vi "DOE Add TC Calibration.vi"(7 "Enum":T1, 10 "TC Coefficients":T2, 11 "Non Cal Temp":dbl) -> (3 "Calibrated Temp":dbl)   [LabVIEW 2014]
uses:
  Utility/Type Definitions/UTILITY TC Coefficients.ctl
  Type Definitions/DOE TC Coefficients Selector.ctl
panel:
  out "output variable":dbl
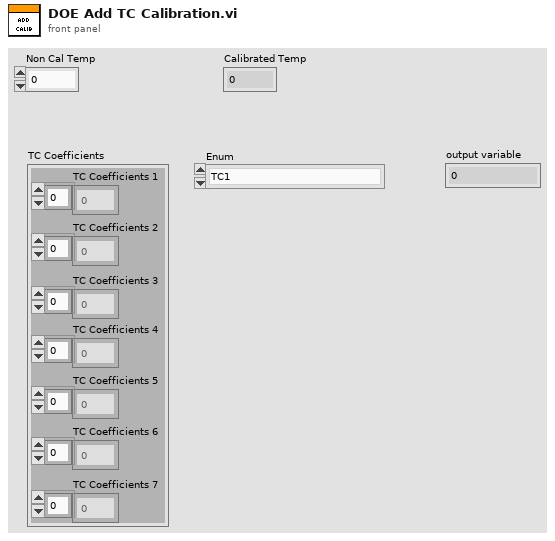
[diagram p1: front panel]
types:
  T1 = typedef "DOE TC Coefficients Selector.ctl" = enum16{"TC1", "TC2", "TC3", "TC4", "TC5", "TC6", "TC7"}
  T2 = typedef "UTILITY TC Coefficients.ctl" = cluster{"TC Coefficients 1":dbl[], "TC Coefficients 2":dbl[], "TC Coefficients 3":dbl[], "TC Coefficients 4":dbl[], "TC Coefficients 5":dbl[], "TC Coefficients 6":dbl[], "TC Coefficients 7":dbl[]}
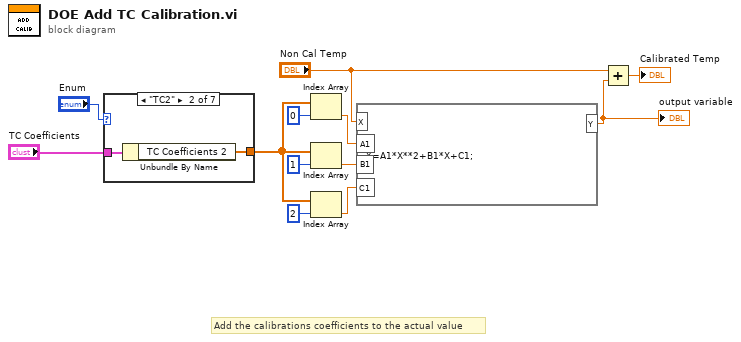
[diagram p0: block diagram]
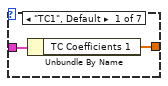
[diagram p2: hidden frame]
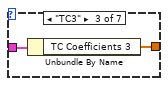
[diagram p3: hidden frame]
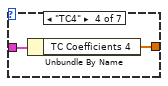
[diagram p4: hidden frame]
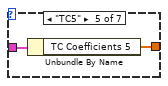
[diagram p5: hidden frame]
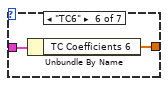
[diagram p6: hidden frame]
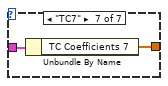
[diagram p7: hidden frame]
diagram:
  # "Add the calibrations coefficients to the actual value"
  n1 = case shown="\"TC2\"" "Enum" {
    tunnel: [w14 w15 w17 w19 w21 w23 w25] -> w3
    tunnel: "TC Coefficients" -> [w13 w16 w18 w20 w22 w24 w26]
    frame "TC1", Default {
      n2 = Unbundle By Name(w13) -> ("TC Coefficients 1"=w14:dbl[])
    }
    frame "TC2" {
      n3 = Unbundle By Name(w16) -> ("TC Coefficients 2"=w15:dbl[])
    }
    frame "TC3" {
      n4 = Unbundle By Name(w18) -> ("TC Coefficients 3"=w17:dbl[])
    }
    frame "TC4" {
      n5 = Unbundle By Name(w20) -> ("TC Coefficients 4"=w19:dbl[])
    }
    frame "TC5" {
      n6 = Unbundle By Name(w22) -> ("TC Coefficients 5"=w21:dbl[])
    }
    frame "TC6" {
      n7 = Unbundle By Name(w24) -> ("TC Coefficients 6"=w23:dbl[])
    }
    frame "TC7" {
      n8 = Unbundle By Name(w26) -> ("TC Coefficients 7"=w25:dbl[])
    }
  }
  n9 = Index Array(array=w3, index=0) -> (element=w7:dbl)
  n10 = Index Array(array=w3, index=1) -> (element=w8:dbl)
  n11 = Index Array(array=w3, index=2) -> (element=w9:dbl)
  n12 = formula code="Y=A1*X**2+B1*X+C1;"("X"="Non Cal Temp", "A1"=w7, "B1"=w8, "C1"=w9) -> ("Y"=w11:dbl)
  "output variable" <- w11
  n13 = Add(x="Non Cal Temp", y=w11) -> (x+y=→"Calibrated Temp":dbl)
